vi "getAzimuth.vi"(8 "error in (no error)":errorcluster, 11 "DomeController in":refnum<class "DomeController.lvclass">) -> (0 "error out":errorcluster, 2 "azimuth":T1 min=0.0 max=360.0, 3 "DomeController out":refnum<class "DomeController.lvclass">)   [LabVIEW 2016, in "DomeController.lvclass"]
uses:
  DomeController.lvclass
  IDome/domeTypedefs/azimuth.ctl
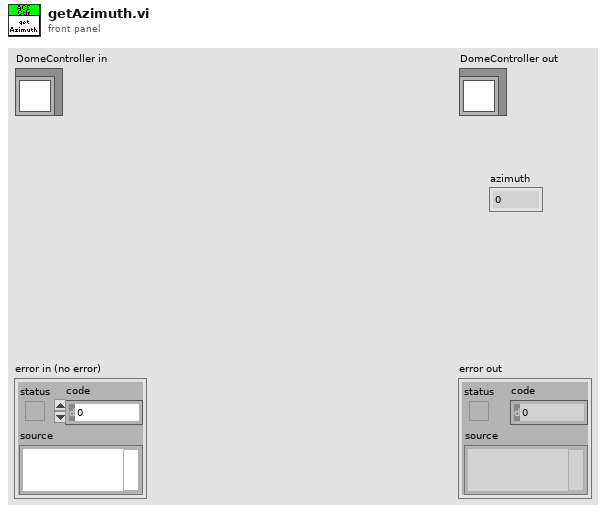
[diagram p1: front panel]
types:
  T1 = typedef "azimuth.ctl" = dbl
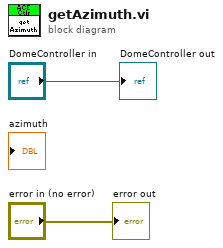
[diagram p0: block diagram]
diagram:
  "error out" <- "error in (no error)"
  "DomeController out" <- "DomeController in"
